vi "Update Load dU Values.vi"(0 "Heat Flow Results in":refnum<class "Heat Flow Results.lvclass">, 5 "R load U":dbl, 7 "I Load":dbl, 9 "P_teg":dbl, 11 "error in":errorcluster) -> (4 "Heat Flow Results out":refnum<class "Heat Flow Results.lvclass">, 15 "error out":errorcluster)   [LabVIEW 2019, in "Results.lvlib" / "Heat Flow Results.lvclass"]
uses:
  Heat Flow Results.lvclass
  Heat Flow Results.lvclass/Heat Flow Results.ctl
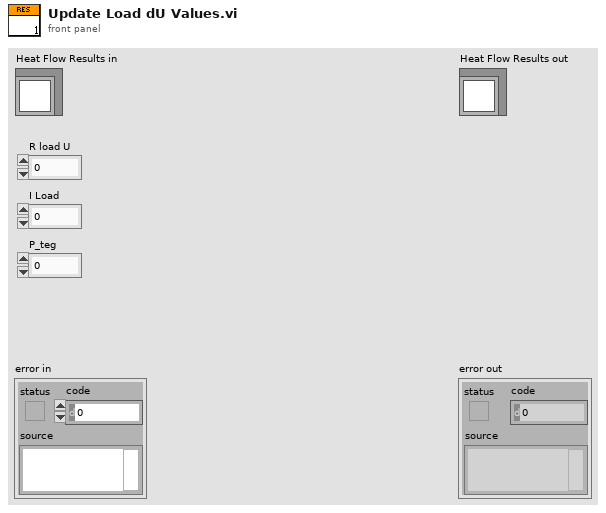
[diagram p1: front panel]
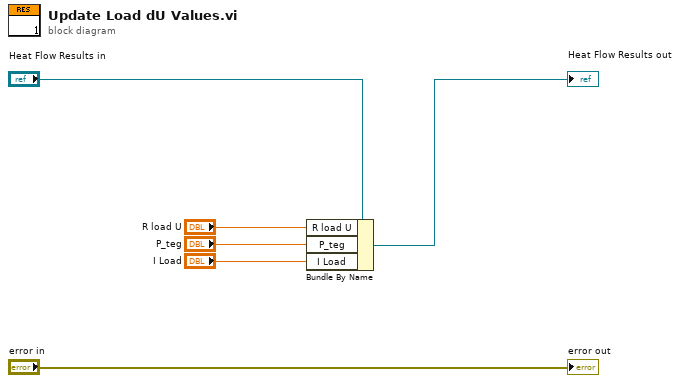
[diagram p0: block diagram]
diagram:
  n1 = Bundle By Name(cluster="Heat Flow Results in", "R load U"="R load U", "P_teg"="P_teg", "I Load"="I Load") -> (→"Heat Flow Results out":refnum<class "Heat Flow Results.lvclass">)
  "error out" <- "error in"
